vi "VISA.vi"(8 "error in (no error)":errorcluster, 10 "string to write":string, 11 "Cobolt in":refnum<class "Cobolt.lvclass">) -> (0 "error out":errorcluster, 2 "buffer out":string, 3 "Cobolt out":refnum<class "Cobolt.lvclass">)   [LabVIEW 2012, in "Cobolt.lvclass"]
uses:
  Cobolt.lvclass
  Cobolt.lvclass/Cobolt.ctl
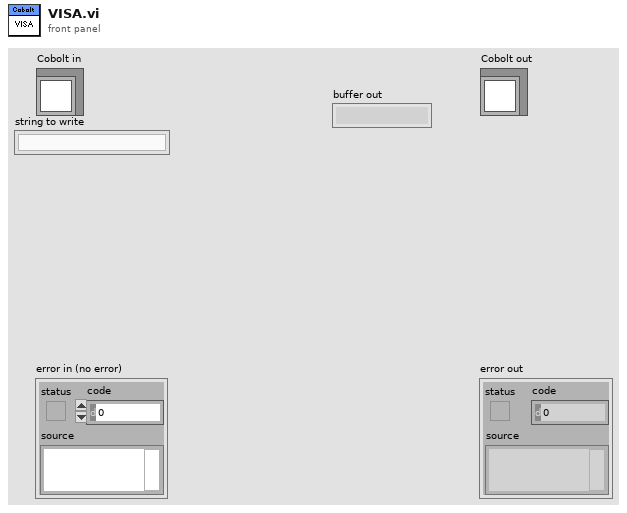
[diagram p1: front panel]
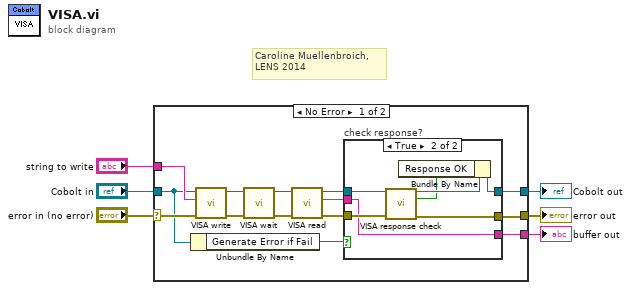
[diagram p0: block diagram]
diagram:
  # "Caroline Muellenbroich, \nLENS 2014"
  n1 = case shown="No Error" "error in (no error)" {
    selector: "error in (no error)" -> [w18 w32]
    tunnel: [w12 w32] -> w5
    tunnel: [w11 w31] -> w3
    tunnel: "Cobolt in" -> [w9 w31]
    tunnel: "string to write" -> [w15 _]
    tunnel: [w7 _] -> w1
    frame No Error {
      n2 = Unbundle By Name(w9) -> ("Generate Error if Fail"=w8:bool)
      n3 = call-dynamic "VISA write.vi"("error in (no error)"=w18, "stringtowrite"=w15, "Cobolt in"=w9) -> ("error out"=w17:errorcluster, "Cobolt out"=w20:refnum<class "Cobolt.lvclass">)  [unwired: 7 in]
      n4 = call-dynamic "VISA wait.vi"("error in (no error)"=w17, "Cobolt in"=w20) -> ("error out"=w16:errorcluster, "Cobolt out"=w19:refnum<class "Cobolt.lvclass">)  [unwired: 8 in]
      n5 = call-dynamic "VISA read.vi"("error in (no error)"=w16, "Cobolt in"=w19) -> ("error out"=w13:errorcluster, "buffer out"=w10:string, "Cobolt out"=w14:refnum<class "Cobolt.lvclass">)  [unwired: 7 in]
      n6 = case "check response?" shown="True" w8 {
        tunnel: w14 -> [w22 w30]
        tunnel: w13 -> [w23 w29]
        tunnel: [w23 w28] -> w12
        tunnel: [w22 w25] -> w11
        tunnel: w10 -> [w21 w27]
        tunnel: [w21 w27] -> w7
        frame False {
        }
        frame True {
          n7 = call-dynamic "VISA response check.vi"("Cobolt in"=w30, "error in (no error)"=w29) -> ("Cobolt out"=w26:refnum<class "Cobolt.lvclass">, "ResponseOK"=w24:bool, "error out"=w28:errorcluster)  [unwired: 10 in, 1 out]
          n8 = Bundle By Name(cluster=w26, "Response OK"=w24) -> (w25:refnum<class "Cobolt.lvclass">)
        }
      }
    }
    frame Error {
    }
  }
  "error out" <- w5
  "Cobolt out" <- w3
  "buffer out" <- w1
